vi "SetExternalInterfaces.vi"(8 "ErrorIn":errorcluster, 10 "ExternalInterfaces":T1[](array[typedef]), 11 "ObjectIn":refnum<class "YAFTAF.lvclass">) -> (0 "ErrorOut":errorcluster, 3 "ObjectOut":refnum<class "YAFTAF.lvclass">)   [LabVIEW 2021, in "YAFTAF.lvclass"]
uses:
  YAFTAF.lvclass
  C:/Localdata/Projects/TriekselSoft/TriekselsoftApplicationFramework/Source/.Externals/Library_YAF/YActor/YActor.lvclass
  Library_TAF_Support/ClusterArrayConversion/BundledArray.ctl
  YActor/YActor.lvclass/YActor.ctl
  YActor/ExeCmd_sync.vi
  YActor/private/SendCommand.vi
  YActor/private/WaitForReply.vi
  YActor/private/CreateLocalVI.vi
  YActor/private/ExeuteInlineVI.vi
  YActor/private/GetRemoteVIRef.vi
  YActor/private/GetNameOfVI.vi
  YActor/QuickCast.vi
  YActor/private/VINameProperty.vi
  YActor/private/MessageCounter.vi
  YActor/InlineReferencePool.vi
  YActor/private/ExecuteVI.vi
  YActor/YActor.lvclass
  YAFTAF.lvclass/YAFTAF.ctl
  C:/Localdata/Projects/TriekselSoft/TriekselsoftApplicationFramework/Source/.Externals/Interface_UserInterface_IFrontPanel/IFrontPanel/IFrontPanel.lvclass
  C:/Localdata/Projects/TriekselSoft/TriekselsoftApplicationFramework/Source/IInterface/IInterface.lvclass
  C:/Localdata/Projects/TriekselSoft/TriekselsoftApplicationFramework/Source/.Externals/Interface_Object_ICreateDestroy/ICreateDestroy/ICreateDestroy.lvclass
  C:/Localdata/Projects/TriekselSoft/TriekselsoftApplicationFramework/Source/.Externals/Interface_Object_IPersistentData/IPersistentData/IPersistentData.lvclass
  C:/Localdata/Projects/TriekselSoft/TriekselsoftApplicationFramework/Source/.Externals/Interface_TAF_ITAFObject/ITAFObject/ITAFObject.lvclass
  C:/Localdata/Projects/TriekselSoft/TriekselsoftApplicationFramework/Source/.Externals/Library_YAF/YAFTAF/YAFTAF.lvclass
  Library_TAF_Support/ClusterArrayConversion/ClusterArrayConversion.lvlib
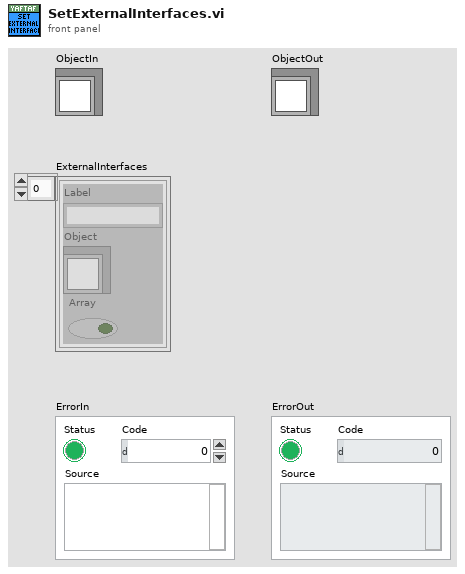
[diagram p1: front panel]
types:
  T1 = typedef "ClusterArrayConversion.lvlib/BundledArray.ctl" = cluster{"Label":string, "Object":refnum<class>, "Array":bool}
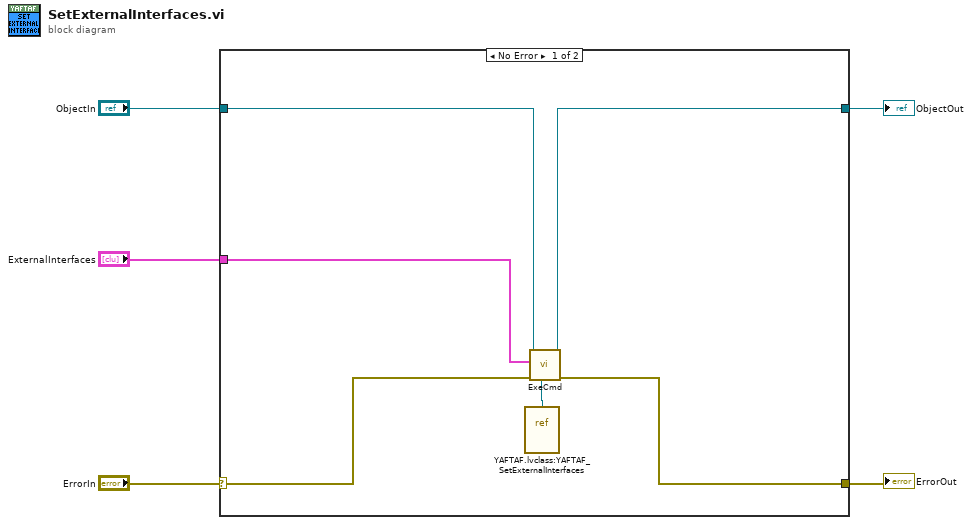
[diagram p0: block diagram]
diagram:
  n1 = case shown="No Error" "ErrorIn" {
    selector: "ErrorIn" -> [w10 w13]
    tunnel: [w11 w13] -> w4
    tunnel: [w8 w12] -> w2
    tunnel: "ObjectIn" -> [w6 w12]
    tunnel: "ExternalInterfaces" -> [w7 _]
    frame No Error {
      n2 = vi-ref "YAFTAF.lvclass:YAFTAF_SetExternalInterfaces.vi"() -> (w9:refnum<vi>)
      n3 = call-poly "ExeCmd.vi"("CmdVIRef"=w9, "ErrorIn"=w10, "CmdData"=w7, "YActorIn"=w6) -> ("ErrorOut"=w11:errorcluster, "YActorOut"=w8:refnum<class "YAFTAF.lvclass">)  [unwired: 5 in, 1 out]
    }
    frame Error {
    }
  }
  "ErrorOut" <- w4
  "ObjectOut" <- w2
